vi "Euler 003.vi"() -> ()   [LabVIEW 2021]
uses:
  <vilib>/gmath/NI_AAL_MathFunc.lvlib
panel:
  out "Largest Prime Factor":i32
  out "Prime Factors Brute":i32[](array[numeric])
  out "Prime Factors by Function":i32[](array[numeric])
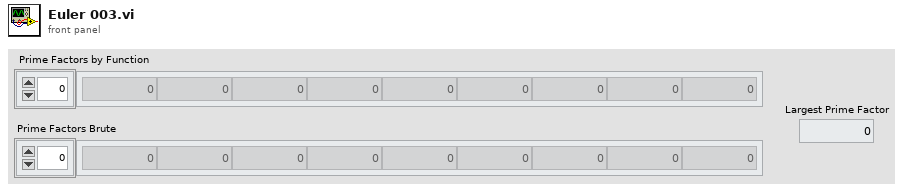
[diagram p1: front panel]
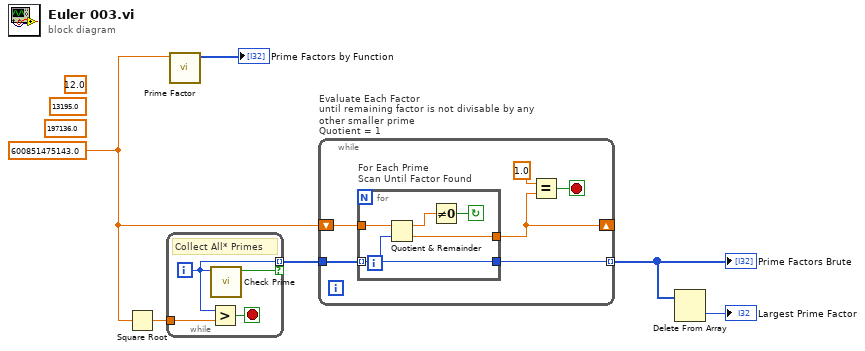
[diagram p0: block diagram]
diagram:
  (unwired) 197136.0
  w3 = 600851475143.0
  (unwired) 13195.0
  (unwired) 12.0
  n1 = Square Root(x=w3) -> (sqrt(x)=w5:dbl)
  n2 = while {
    tunnel: w5 -> [w10]
    tunnel: [w9] -> w4 mode=indexing if=w8
    i -> [w9]
    stop <- w7 stop-if-true
    # "Collect All* Primes"
    n3 = Greater?(x=w9, y=w10) -> (0:w7:bool)
    n4 = call <vilib>:"Check Prime.vi"("n"=w9) -> ("prime?"=w8:bool)  [unwired: 10 in]
  }
  n5 = call <vilib>:"Prime Factor.vi"("n"=w3) -> ("Prime Factors"=→"Prime Factors by Function":i64[])  [unwired: 9 in]
  n6 = while "Evaluate Each Factor \nuntil remaining factor is not divisable by any other smaller prime\nQuotient = 1" {
    tunnel: w4 -> [w16]
    shift-right: [w13] -> _
    shift-left: w3 -> [w15]
    tunnel: [w14] -> w1 mode=indexing
    stop <- w11 stop-if-true
    n7 = for "For Each Prime \nScan Until Factor Found" {
      tunnel: w16 -> [w18] mode=indexing
      tunnel: w15 -> [w20]
      tunnel: [w19] -> w13
      tunnel: [w18] -> w14
      stop <- w17 continue-if-true
      n8 = Quotient & Remainder(x=w20, y=w18) -> (x-y*floor(x/y)=w21:dbl, floor(x/y)=w19:dbl)
      n9 = Not Equal To 0?(x=w21) -> (x != 0?=w17:bool)
    }
    n10 = Equal?(x=1.0 ("y"), y=w13) -> (x = y?=w11:bool)
  }
  "Prime Factors Brute" <- w1
  n11 = Delete From Array(array=w1) -> (deleted portion=→"Largest Prime Factor":i32)  [unwired: 2 in, 1 out]
